vi "Creat Fits.vi"(8 "error in (no error)":errorcluster, 11 "CCDCamera in":refnum<class "CCDCamera.lvclass">) -> (0 "error out":errorcluster, 3 "CCDCamera out":refnum<class "CCDCamera.lvclass">)   [LabVIEW 2018, in "CCDCamera.lvclass"]
doc: "Este VI cria um arquivo FITS contendo a última imagem obtida."
uses:
  CCDCamera.lvclass
  <userlib>/gfitsio/cfitsio-bitpix.ctl
  CCDCamera.lvclass/CCDCamera.ctl
  <userlib>/gfitsio/gfitsio-write-image-subset-dbl-2d.vi
  <userlib>/gfitsio/gfitsio.lvlib
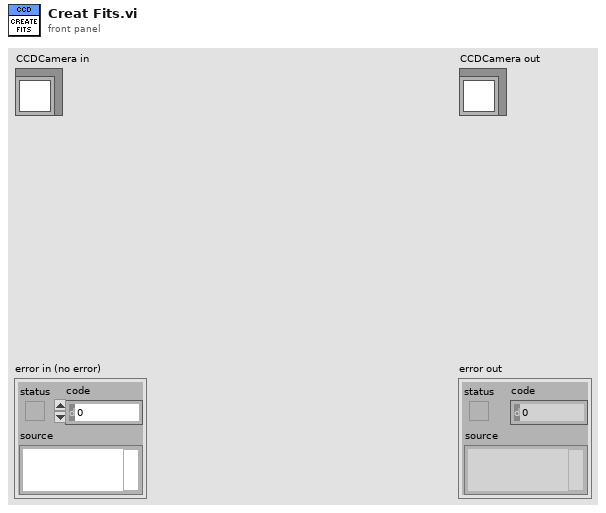
[diagram p1: front panel]
types:
  T1 = enum16{"open", "open or create", "create or replace", "create", "open (read only)"}
  T2 = enum16{"open", "open or create", "create", "create or replace"}
  T3 = typedef "gfitsio.lvlib/cfitsio-bitpix.ctl" = i32
  T4 = typedef "gfitsio.lvlib/gfitsio-refnum.ctl" = refnum<k1>
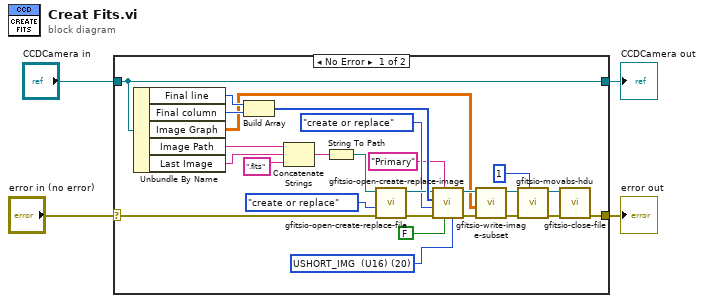
[diagram p0: block diagram]
diagram:
  n1 = case shown="No Error" "error in (no error)" {
    selector: "error in (no error)" -> [w23 w32]
    tunnel: [w22 w32] -> w3
    tunnel: [w30 w31] -> w1
    tunnel: "CCDCamera in" -> [w30 w31]
    frame No Error {
      w14 = T3 20 items=["<invalid type>"=0, "BYTE_IMG  (U8)"=8, "SHORT_IMG  (I16)"=16, "USHORT_IMG  (U16)"=20, "LONG_IMG  (I32)"=32, "ULONG_IMG  (U32)"=40, "FLOAT_IMG  (SGL)"=-32, "DOUBLE_IMG  (DBL)"=-64] ("image data type")
      n2 = Unbundle By Name(w30) -> ("Final line"=w28:u32, "Final column"=w29:u32, "Image Graph"=w13:dbl[][], "Image Path"=w11:string, "Last Image"=w10:string)
      n3 = Build Array(w28, w29) -> (w21:u32[])
      n4 = Concatenate Strings(w11, w10, ".fits") -> (w8:string)
      n5 = String To Path(string=w8) -> (path=w7:path)
      n6 = call <userlib>:"gfitsio-open-create-replace-file.vi"("error in (no error)"=w23, "function (open)"=T1."create or replace", "file path (dialog if empty)"=w7) -> ("error out"=w27:errorcluster, "gfits refnum"=w20:T4)  [unwired: 6 in, 1 out]
      n7 = call <userlib>:"gfitsio-open-create-replace-image.vi"("image data type"=w14, "advisory dialog? (display:T)"=FALSE, "hdu name (dialog if empty)"="Primary" ("prompt"), "error in (no error)"=w27, "function (open or create)"=T2."create or replace", "naxes"=w21, "gfits refnum"=w20) -> ("error out"=w26:errorcluster, "dup gfits refnum"=w19:T4)  [unwired: 2 in, 1 out]
      n8 = call-poly <userlib>:"gfitsio-write-image-subset.vi"("error in (no error)"=w26, "data"=w13, "gfits refnum"=w19) -> ("error out"=w25:errorcluster, "dup gfits refnum"=w18:T4)  [unwired: 7 in]
      n9 = call <userlib>:"gfitsio-movabs-hdu.vi"("hdunum"=1, "error in (no error)"=w25, "gfits refnum"=w18) -> ("error out"=w24:errorcluster, "dup gfits refnum"=w17:T4)  [unwired: 6 in, 1 out]
      n10 = call <userlib>:"gfitsio-close-file.vi"("error in (no error)"=w24, "gfits refnum"=w17) -> ("error out"=w22:errorcluster)  [unwired: 8 in, 1 out]
    }
    frame Error {
    }
  }
  "error out" <- w3
  "CCDCamera out" <- w1
